vi "Multi Functional Global Variable 2012 NIVerified.vi"() -> ()   [LabVIEW 2012]
panel:
  in  "stop":bool
  in  "Number In":dbl
  in  "String In":string
  out "Elapsed Time Out":dbl
  out "Number Out":dbl
  out "String Out":string
  out "Read Elapsed Time":dbl
  out "Read Number":dbl
  out "Read String":string
  in  "Operation":T1(ring)
  # "Overview: This example demonstrates how to create multiple Functional Global Variables and use them in an application.\nRequirements: LabVIEW Base Development System 2012 or compatible\nInstructions:\n1- Run the VI\n2- Use the Operation control to select the desired action (Set String, Set Numeric, Reset Time)\n3- Test the stored values by changing the Operation control to (Get String, Get Numeric, Get Elapsed Time)"
  # "Values from Read Only Loop"
  # "Control Multi-Functional Global"
  # "Values from Read/Write Loop"
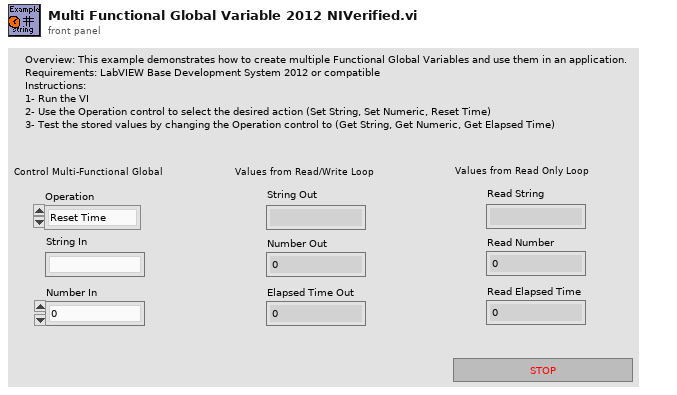
[diagram p1: front panel]
types:
  T1 = enum16{"Reset Time", "Set String", "Set Number", "Get Elapsed Time", "Get String", "Get Number"}
  T2 = cluster{"Operation":enum16{"Reset Time", "Set String", "Set Number", "Get Elapsed Time", "Get String", "Get Number"}, "Data":variant}
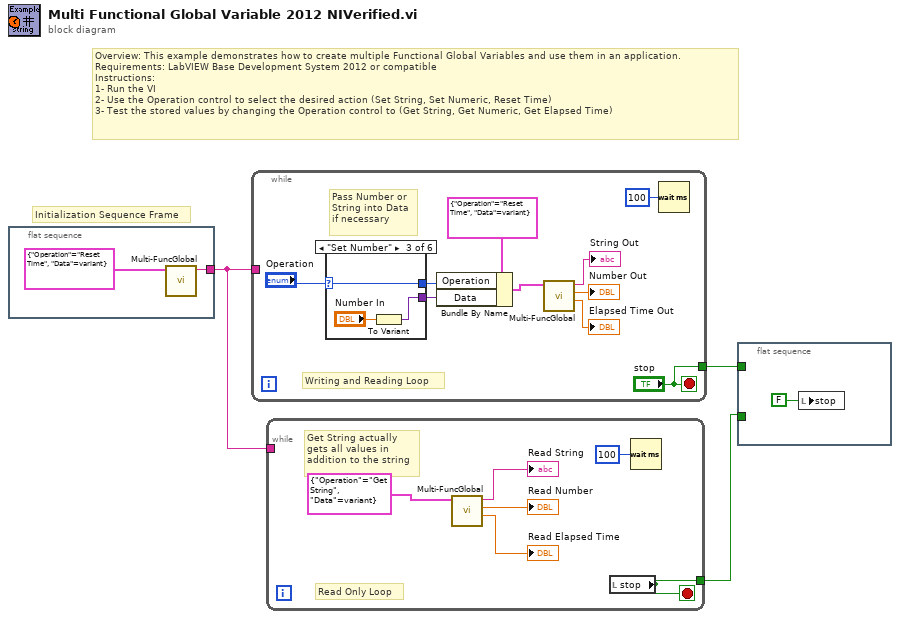
[diagram p0: block diagram]
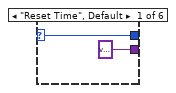
[diagram p2: hidden frame]
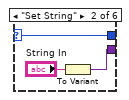
[diagram p3: hidden frame]
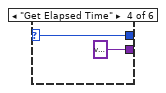
[diagram p4: hidden frame]
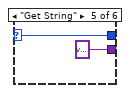
[diagram p5: hidden frame]
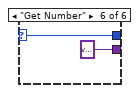
[diagram p6: hidden frame]
diagram:
  # "Overview: This example demonstrates how to create multiple Functional Global Variables and use them in an application.\nRequirements: LabVIEW Base Development System 2012 or compatible\nInstructions:\n1- Run the VI\n2- Use the Operation control to select the desired action (Set String, Set Numeric, Reset Time)\n3- Test the stored values by changing the Operation control to (Get String, Get Numeric, Get Elapsed Time)"
  # "Initialization Sequence Frame"
  n1 = flat-sequence {
    tunnel: [w4] -> w3
    frame #0 {
      n2 = call "Multi-FuncGlobal.vi"("Operation and Data In"=T2 {"Operation"=enum."Reset Time", "Data"=variant}) -> ("String Out"=w4:string)  [unwired: 10 out]
    }
  }
  n3 = while {
    tunnel: w3 -> [_]
    tunnel: ["stop"] -> w1
    stop <- "stop" stop-if-true
    # "Pass Number or\nString into Data\nif necessary"
    # "Writing and Reading Loop"
    n4 = case shown="\"Set Number\"" "Operation" {
      selector: "Operation" -> [w17 w20 w23 w25 w27 w29]
      tunnel: [w17 w20 w23 w25 w27 w29] -> w8
      tunnel: [variant ("Variant") w18 w21 variant ("Variant") variant ("Variant") variant ("Variant")] -> w7
      frame "Reset Time", Default {
      }
      frame "Set String" {
        n5 = To Variant(anything="String In") -> (Variant=w18:variant)
      }
      frame "Set Number" {
        n6 = To Variant(anything="Number In") -> (Variant=w21:variant)
      }
      frame "Get Elapsed Time" {
      }
      frame "Get String" {
      }
      frame "Get Number" {
      }
    }
    n7 = Bundle By Name(cluster=T2 {"Operation"=enum."Reset Time", "Data"=variant} ("Operation and Data In"), "Operation"=w8, "Data"=w7) -> (w13:T2)
    n8 = call "Multi-FuncGlobal.vi"("Operation and Data In"=w13) -> ("Time Out"=→"Elapsed Time Out":dbl, "Numeric Out"=→"Number Out":dbl, "String Out"=→"String Out":string)  [unwired: 8 out]
    n9 = Wait (ms)(milliseconds to wait=u32 100) -> ()  [unwired: 1 out]
  }
  n10 = while {
    tunnel: w3 -> [_]
    tunnel: [w30] -> w2
    stop <- w30 stop-if-true
    # "Get String actually\ngets all values in \naddition to the string"
    # "Read Only Loop"
    n11 = call "Multi-FuncGlobal.vi"("Operation and Data In"=T2 {"Operation"=enum."Get String", "Data"=variant}) -> ("Time Out"=→"Read Elapsed Time":dbl, "Numeric Out"=→"Read Number":dbl, "String Out"=→"Read String":string)  [unwired: 8 out]
    n12 = local read "stop"() -> (w30:bool)
    n13 = Wait (ms)(milliseconds to wait=u32 100) -> ()  [unwired: 1 out]
  }
  n14 = flat-sequence {
    tunnel: w2 -> [_]
    tunnel: w1 -> [_]
    frame #0 {
      n15 = local write "stop"(FALSE ("stop")) -> ()
    }
  }
